vi "Error List Editor.vi"() -> ()   [LabVIEW 2020]
uses:
  Error Description.ctl
panel:
  in  "Path":path
  in  "Delete":bool
  in  "Add":bool
  in  "Close":bool
  in  "Undo":bool
  in  "Save":bool
  in  "Details":string
  in  "Description":string
  in  "Code":i32(listbox)
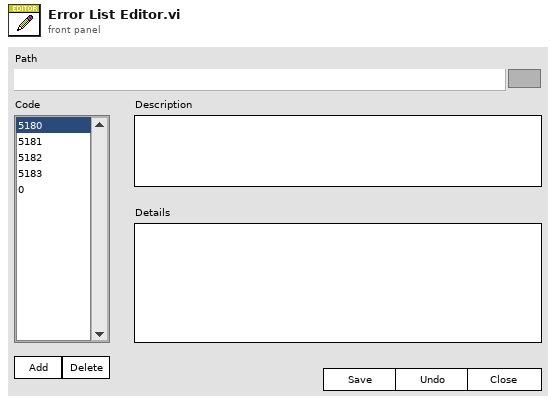
[diagram p1: front panel]
types:
  T1 = enum8{"Enabled", "Disabled", "Disabled and Grayed Out"}
  T2 = typedef "Error Description.ctl" = cluster{"Code":i32, "Description":string, "Details":string}
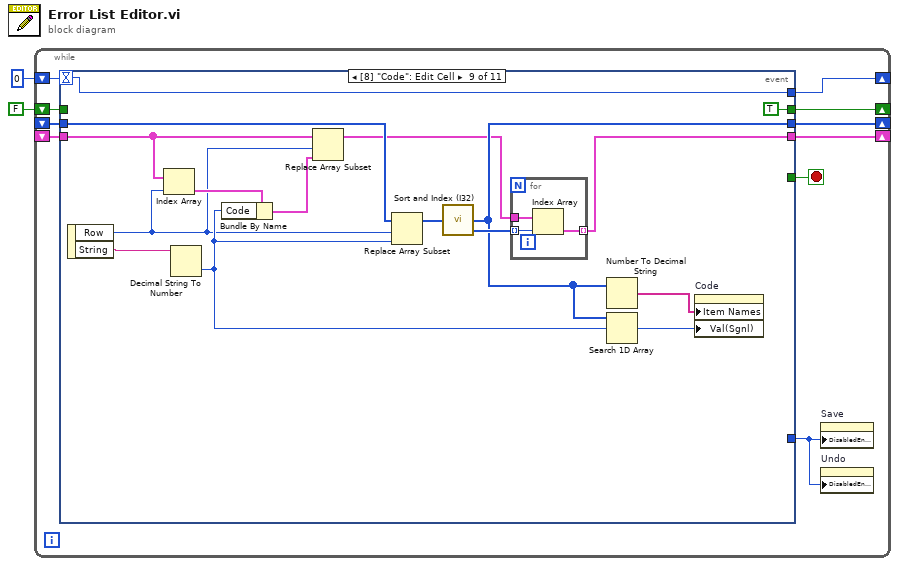
[diagram p0: block diagram]
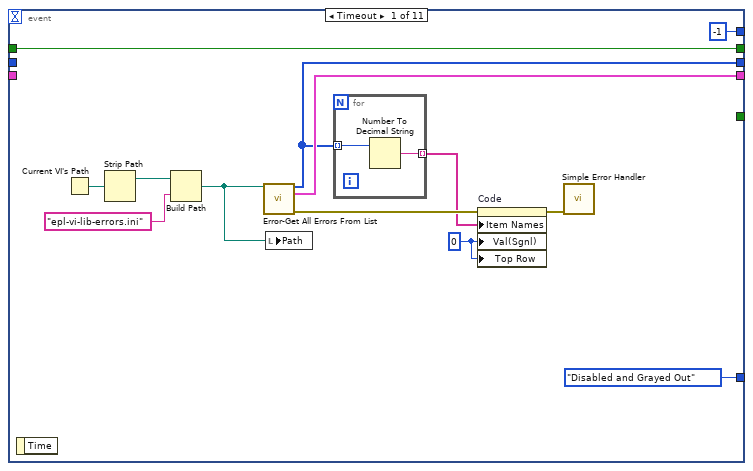
[diagram p2: hidden frame]
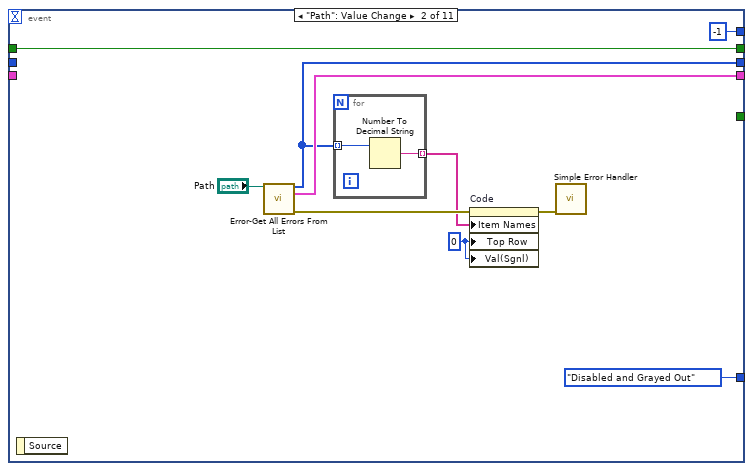
[diagram p3: hidden frame]
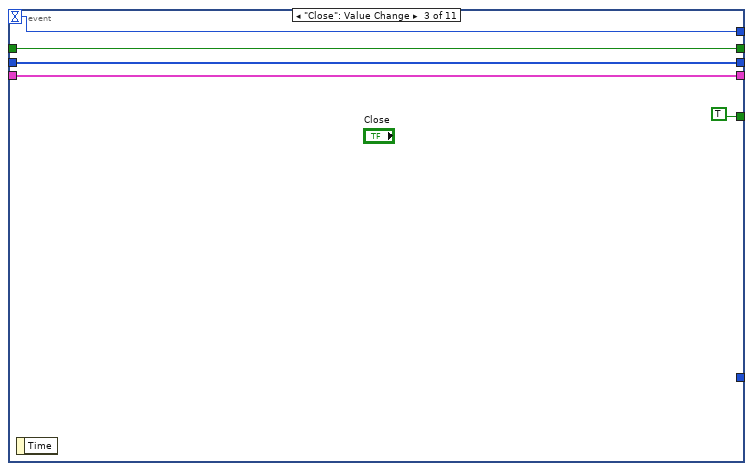
[diagram p4: hidden frame]
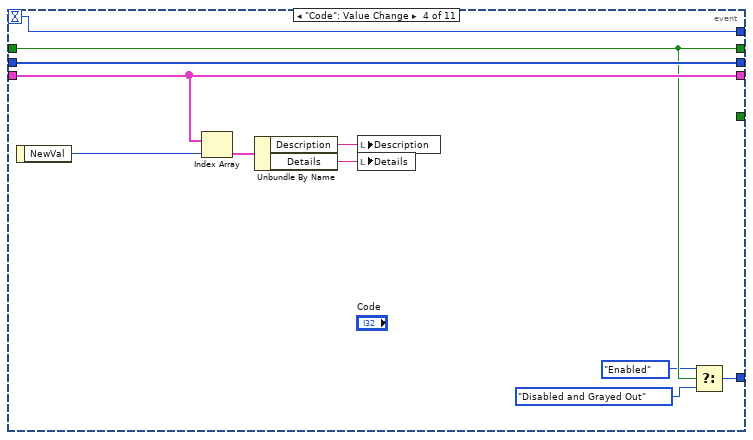
[diagram p5: hidden frame]
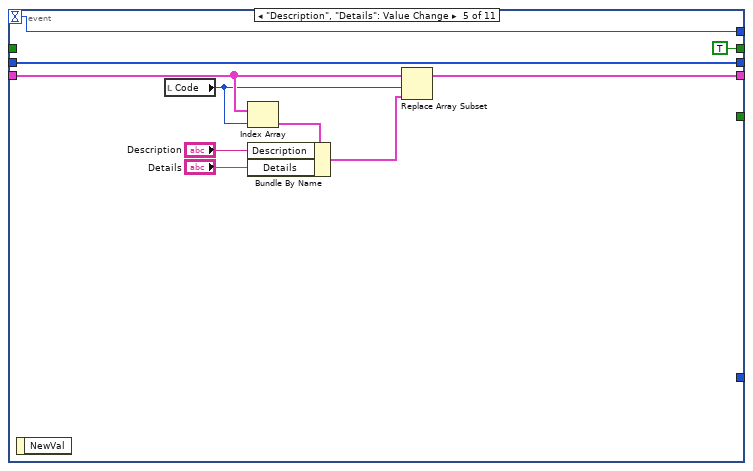
[diagram p6: hidden frame]
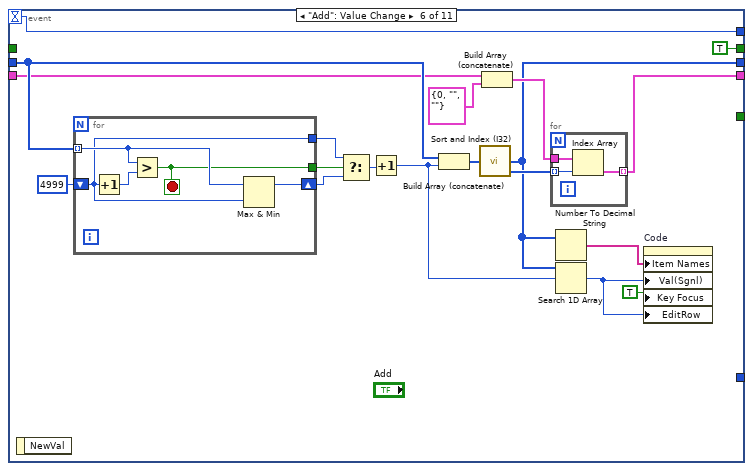
[diagram p7: hidden frame]
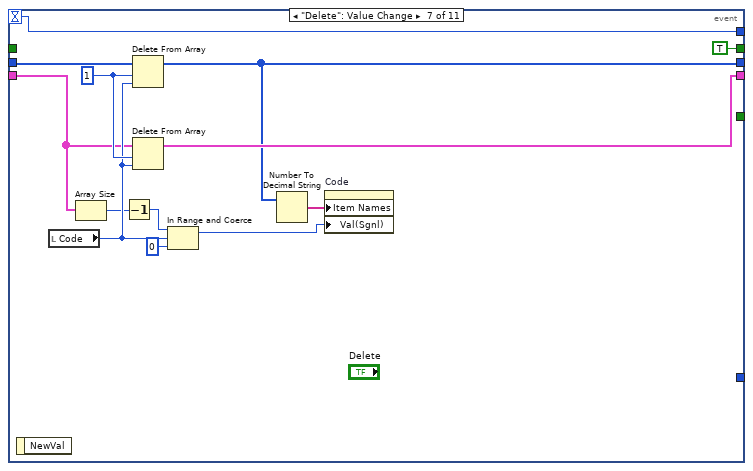
[diagram p8: hidden frame]
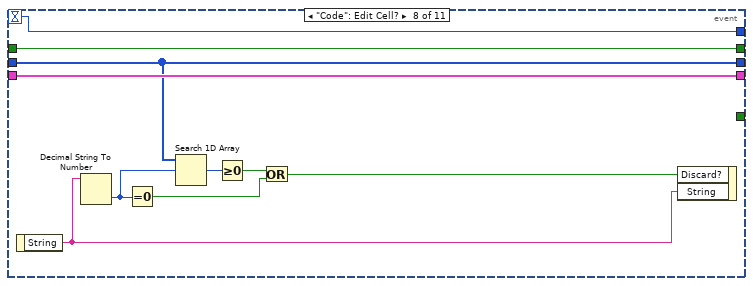
[diagram p9: hidden frame]
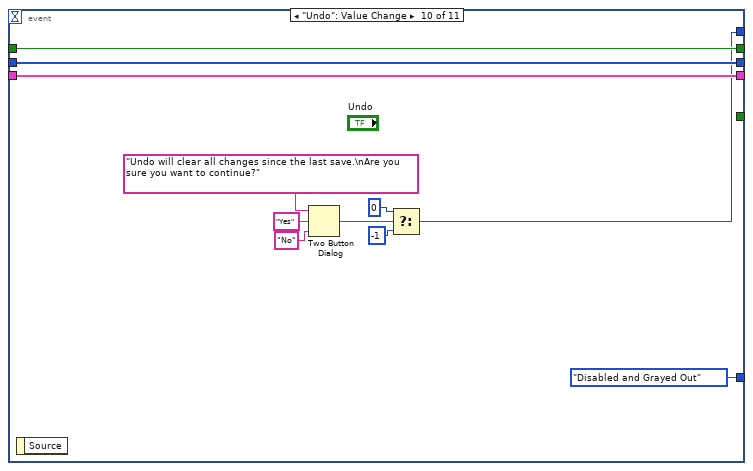
[diagram p10: hidden frame]
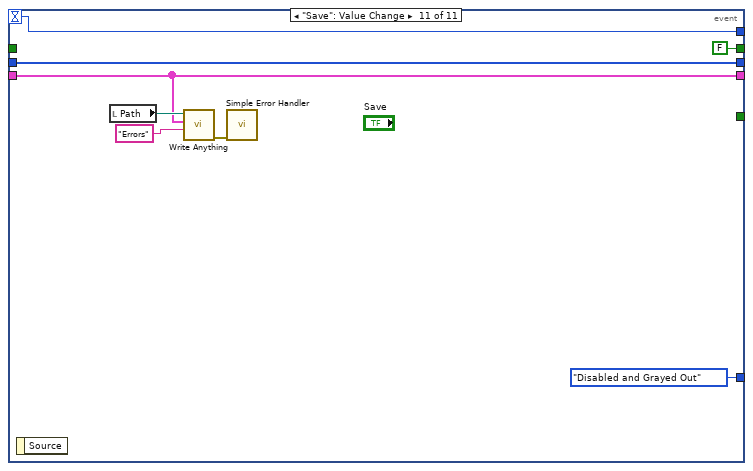
[diagram p11: hidden frame]
diagram:
  n1 = while {
    shift-right: [w11] -> _
    shift-left: 0 -> [w12]
    shift-right: [w8] -> _
    shift-left: FALSE -> [w9]
    shift-right: [w7] -> _
    shift-left: _ -> [w6]
    shift-right: [w5] -> _
    shift-left: _ -> [w4]
    stop <- w10 stop-if-true
    n2 = event shown="[8] \"Code\": Edit Cell" {
      selector: _ -> [_ _ _ _ _ _ _ _ _ _ _]
      dyn-events: _ -> [_ _ _ _ _ _ _ _ _ _ _]
      timeout: w12 -> [_ _ w44 w55 w65 w84 w105 w115 w131 _ w152]
      tunnel: [-1 -1 w44 w55 w65 w84 w105 w115 w131 w136 w152] -> w11
      tunnel: [_ _ TRUE _ _ _ _ _ _ _ _] -> w10
      tunnel: [w24 w36 w42 w48 TRUE TRUE TRUE w114 TRUE w145 FALSE] -> w8
      tunnel: w9 -> [w24 w36 w42 w48 _ _ _ w114 _ w145 _]
      tunnel: [w21 w33 w41 w54 w57 w73 w101 w113 w123 w143 w148] -> w7
      tunnel: w6 -> [_ _ w41 w54 w60 w77 w96 w113 w121 w143 w148]
      tunnel: [w19 w31 w40 w50 w56 w71 w99 w112 w122 w144 w150] -> w5
      tunnel: w4 -> [_ _ w40 w50 w56 w78 w102 w112 w129 w144 w150]
      tunnel: [T1."Disabled and Grayed Out" ("Disabled") T1."Disabled and Grayed Out" ("Disabled") _ w49 _ _ _ _ _ T1."Disabled and Grayed Out" ("Disabled") T1."Disabled and Grayed Out" ("Disabled")] -> w3
      event Timeout {
        w13 = 0 ("Value (Signaling)")
        n3 = event-data() -> ()  [unwired: 1 in, 1 out]
        n4 = Current VI's Path() -> (path=w16:path)
        n5 = Strip Path(path=w16) -> (stripped path=w17:path)  [unwired: 1 out]
        n6 = Build Path(base path=w17, name or relative path="epl-vi-lib-errors.ini") -> (appended path=w14:path)
        n7 = call "Error-Get All Errors From List.vi"("Path"=w14) -> ("Codes"=w19:i32[], "Errors"=w21:T2[], "error out"=w23:errorcluster)  [unwired: 12 in]
        n8 = local write "Path"(w14) -> ()
        n9 = for {
          tunnel: w19 -> [w27] mode=indexing
          tunnel: [w26] -> w18 mode=indexing
          n10 = Number To Decimal String(number=w27) -> (decimal integer string=w26:string)  [unwired: 1 in]
        }
        n11 = property on="Code" class="LstBox (strict)"(error in=w23, "Item Names"=w18, "Val(Sgnl)"=w13, "Top Row"=w13) -> (error out=w22:errorcluster)  [unwired: 1 in, 1 out]
        n12 = call <vilib>:"Simple Error Handler.vi"("error in (no error)"=w22) -> ()  [unwired: 4 in, 5 out]
      }
      event "Path": Value Change {
        w28 = 0 ("Value (Signaling)")
        n13 = event-data() -> ()  [unwired: 1 in, 1 out]
        n14 = call "Error-Get All Errors From List.vi"("Path"="Path") -> ("Codes"=w31:i32[], "Errors"=w33:T2[], "error out"=w35:errorcluster)  [unwired: 12 in]
        n15 = for {
          tunnel: w31 -> [w39] mode=indexing
          tunnel: [w38] -> w30 mode=indexing
          n16 = Number To Decimal String(number=w39) -> (decimal integer string=w38:string)  [unwired: 1 in]
        }
        n17 = property on="Code" class="LstBox (strict)"(error in=w35, "Item Names"=w30, "Top Row"=w28, "Val(Sgnl)"=w28) -> (error out=w34:errorcluster)  [unwired: 1 in, 1 out]
        n18 = call <vilib>:"Simple Error Handler.vi"("error in (no error)"=w34) -> ()  [unwired: 4 in, 5 out]
      }
      event "Close": Value Change {
        n19 = event-data() -> ()  [unwired: 1 in, 1 out]
      }
      event "Code": Value Change {
        n20 = event-data() -> ("NewVal"=w45:i32)  [unwired: 1 in]
        n21 = Index Array(array=w54, index=w45) -> (element=w53:T2)
        n22 = Unbundle By Name(w53) -> ("Description"=w52:string, "Details"=w51:string)
        n23 = local write "Description"(w52) -> ()
        n24 = local write "Details"(w51) -> ()
        n25 = Select(t=T1."Enabled" ("Disabled"), s=w48, f=T1."Disabled and Grayed Out" ("Disabled")) -> (s? t:f=w49:T1)
      }
      event "Description", "Details": Value Change {
        n26 = event-data() -> ()  [unwired: 1 in, 1 out]
        n27 = local read "Code"() -> (w59:i32)
        n28 = Index Array(array=w60, index=w59) -> (element=w63:T2)
        n29 = Bundle By Name(cluster=w63, "Description"="Description", "Details"="Details") -> (w58:T2)
        n30 = Replace Array Subset(array=w60, new element=w58, index=w59) -> (w57:T2[])
      }
      event "Add": Value Change {
        n31 = event-data() -> ()  [unwired: 1 in, 1 out]
        n32 = for {
          tunnel: w78 -> [w92] mode=indexing
          shift-right: [w90] -> w80
          shift-left: 4999 -> [w88]
          tunnel: [w88] -> w81
          tunnel: [w91] -> w82
          stop <- w91 stop-if-true
          n33 = Increment(x=w88) -> (x+1=w89:i32)
          n34 = Greater?(x=w92, y=w89) -> (0:w91:bool)
          n35 = Max & Min(x=w92, y=w88) -> (max(x,y)=w90:i32)  [unwired: 1 out]
        }
        n36 = Select(t=w81, s=w82, f=w80) -> (s? t:f=w79:i32)
        n37 = Increment(x=w79) -> (x+1=w72:i32)
        n38 = Build Array (concatenate)(w78, w72) -> (w76:i32[])
        n39 = call "Sort and Index (I32).vi"("X"=w76) -> ("Index"=w75:i32[], "Sort(X)"=w71:i32[])  [unwired: 3 in]
        n40 = Build Array (concatenate)(w77, T2 {"Code"=0, "Description"="", "Details"=""} ("error")) -> (w74:T2[])
        n41 = for {
          tunnel: w75 -> [w85] mode=indexing
          tunnel: w74 -> [w87]
          tunnel: [w86] -> w73 mode=indexing
          n42 = Index Array(array=w87, index=w85) -> (element=w86:T2)
        }
        n43 = Number To Decimal String(number=w71) -> (decimal integer string=w70:string[])  [unwired: 1 in]
        n44 = Search 1D Array(1D array=w71, element=w72) -> (index of element=w67:i32)  [unwired: 1 in]
        n45 = property on="Code" class="LstBox (strict)"("Item Names"=w70, "Val(Sgnl)"=w67, "Key Focus"=TRUE, "EditRow"=w67) -> ()  [unwired: 2 in, 2 out]
      }
      event "Delete": Value Change {
        w103 = 1 ("length")
        n46 = event-data() -> ()  [unwired: 1 in, 1 out]
        n47 = local read "Code"() -> (w98:i32)
        n48 = Array Size(array=w96) -> (size(s)=w94:i32)
        n49 = Decrement(x=w94) -> (x-1=w95:i32)
        n50 = Delete From Array(array=w102, length=w103, index=w98) -> (array with subset deleted=w99:i32[])  [unwired: 1 out]
        n51 = Delete From Array(array=w96, length=w103, index=w98) -> (array with subset deleted=w101:T2[])  [unwired: 1 out]
        n52 = In Range and Coerce(upper limit=w95, x=w98, lower limit=0) -> (coerced(x)=w93:i32)  [unwired: 1 out]
        n53 = Number To Decimal String(number=w99) -> (decimal integer string=w100:string[])  [unwired: 1 in]
        n54 = property on="Code" class="LstBox (strict)"("Item Names"=w100, "Val(Sgnl)"=w93) -> ()  [unwired: 2 in, 2 out]
      }
      event "Code": Edit Cell? {
        n55 = event-data() -> ("String"=w106:string)  [unwired: 1 in]
        n56 = Decimal String To Number(string=w106) -> (number=w111:i32)  [unwired: 2 in, 1 out]
        n57 = Equal To 0?(x=w111) -> (x = 0?=w108:bool)
        n58 = Search 1D Array(1D array=w112, element=w111) -> (index of element=w110:i32)  [unwired: 1 in]
        n59 = Greater Or Equal To 0?(x=w110) -> (x >= 0?=w109:bool)
        n60 = Or(x=w109, y=w108) -> (x .or. y?=w107:bool)
        n61 = event-data("Discard?"=w107, "String"=w106) -> ()  [unwired: 1 in, 1 out]
      }
      event "Code": Edit Cell {
        n62 = event-data() -> ("Row"=w116:i32, "String"=w128:string)  [unwired: 1 in]
        n63 = Index Array(array=w121, index=w116) -> (element=w120:T2)
        n64 = Decimal String To Number(string=w128) -> (number=w119:i32)  [unwired: 2 in, 1 out]
        n65 = Bundle By Name(cluster=w120, "Code"=w119) -> (w117:T2)
        n66 = Replace Array Subset(array=w121, new element=w117, index=w116) -> (w118:T2[])
        n67 = Replace Array Subset(array=w129, new element=w119, index=w116) -> (w125:i32[])
        n68 = call "Sort and Index (I32).vi"("X"=w125) -> ("Index"=w124:i32[], "Sort(X)"=w122:i32[])  [unwired: 3 in]
        n69 = for {
          tunnel: w124 -> [w132] mode=indexing
          tunnel: w118 -> [w134]
          tunnel: [w133] -> w123 mode=indexing
          n70 = Index Array(array=w134, index=w132) -> (element=w133:T2)
        }
        n71 = Number To Decimal String(number=w122) -> (decimal integer string=w127:string[])  [unwired: 1 in]
        n72 = Search 1D Array(1D array=w122, element=w119) -> (index of element=w126:i32)  [unwired: 1 in]
        n73 = property on="Code" class="LstBox (strict)"("Item Names"=w127, "Val(Sgnl)"=w126) -> ()  [unwired: 2 in, 2 out]
      }
      event "Undo": Value Change {
        n74 = event-data() -> ()  [unwired: 1 in, 1 out]
        n75 = Two Button Dialog(message="Undo will clear all changes since the last save.\nAre you sure you want to continue?", 1:"No" ("F button name (\"Cancel\")"), 2:"Yes" ("T button name (\"OK\")")) -> (T button?=w139:bool)
        n76 = Select(t=0, s=w139, f=-1) -> (s? t:f=w136:i32)
      }
      event "Save": Value Change {
        n77 = event-data() -> ()  [unwired: 1 in, 1 out]
        n78 = local read "Path"() -> (w149:path)
        n79 = call "Write Anything.vi"("Section Name (Name of \"Anything\")"="Errors" ("Section Name (Name of \"Anything\")"), "Anything"=w148, "Path (dialog)"=w149) -> ("Error Out"=w146:errorcluster)  [unwired: 7 in, 1 out]
        n80 = call <vilib>:"Simple Error Handler.vi"("error in (no error)"=w146) -> ()  [unwired: 4 in, 5 out]
      }
    }
    n81 = property on="Save" class="Bool"("DisabledEnum"=w3) -> ()  [unwired: 2 in, 2 out]
    n82 = property on="Undo" class="Bool"("DisabledEnum"=w3) -> ()  [unwired: 2 in, 2 out]
  }
